vi "Finish.vi"   [LabVIEW 2017]
doc: "This VI is called just before exiting. It is expected to close I/O refnum, save collected data, etc."
uses:
  <vilib>/Rock Robotics/WPI/Utilities/WPI_GetSetVariantRefNum.vi
types:
  T1 = typedef "WPI_MotorControlDeviceRef.ctl" = cluster{"DeviceStatus":errorcluster, "Type":T2, "PWM":cluster{"PWM Channel":T3, "DeadBand":T4}, "CAN":cluster{"Device Number":u8, "SetOutput VI Ref":variant, "GetOutput VI Ref":variant, "Enable VI Ref":variant, "Disable VI Ref":variant, "Data":variant}, "Invert":bool, "DIO PWM":cluster{"PWM \"Enable\" Channel":T3, "DIOChannel":T5, "PWM Rate":dbl}}
  T2 = typedef "WPI_MotorControlType.ctl" = enum16{"PWM", "CAN", "DIO PWM"}
  T3 = typedef "FPGA_DIOPWMChannel.ctl" = enum8{"PWM 0", "PWM 1", "PWM 2", "PWM 3", "PWM 4", "PWM 5", "PWM 6", "PWM 7", "PWM 8", "PWM 9", "PWM MXP 0", "PWM MXP 1", "PWM MXP 2", "PWM MXP 3", "PWM MXP 4", "PWM MXP 5", "PWM MXP 6", "PWM MXP 7", "PWM MXP 8", "PWM MXP 9", "Invalid"}
  T4 = typedef "WPI_PWMDeadband.ctl" = cluster{"Name":string, "maxPositivePwm":i32, "minPositivePwm":i32, "centerPwm":i32, "maxNegativePwm":i32, "minNegativePwm":i32, "angularRange":u16}
  T5 = typedef "FPGA_DIOChannel.ctl" = enum8{"DIO 0", "DIO 1", "DIO 2", "DIO 3", "DIO 4", "DIO 5", "DIO 6", "DIO 7", "DIO 8", "DIO 9", "DIO MXP 0", "DIO MXP 1", "DIO MXP 2", "DIO MXP 3", "DIO MXP 4", "DIO MXP 5", "DIO MXP 6", "DIO MXP 7", "DIO MXP 8", "DIO MXP 9", "DIO MXP 10", "DIO MXP 11", "DIO MXP 12", "DIO MXP 13", "DIO MXP 14", "DIO MXP 15", "SPI Port CS1", "SPI Port CS2", "SPI Port CS3", "SPI Port MISO", "SPI Port MOSI", "Invalid"}
  T6 = typedef "WPI_CompressorDevRef.ctl" = cluster{"DevStatus":errorcluster, "Pneumatics Control Module":u8}
  T7 = typedef "WPI_JoystickDevRef.ctl" = cluster{"Device":T8}
  T8 = typedef "WPI_JoystickDeviceEnum.ctl" = enum16{"USB 0", "USB 1", "USB 2", "USB 3", "USB 4", "USB 5"}
  T9 = typedef "WPI_SolenoidDevRef.ctl" = cluster{"DevStatus":errorcluster, "Pneumatics Control Module":u8, "Forward Solenoid Channel":T10, "Reverse Solenoid Channel":T10}
  T10 = typedef "WPI_SolenoidChannel.ctl" = enum8{"Solenoid 0", "Solenoid 1", "Solenoid 2", "Solenoid 3", "Solenoid 4", "Solenoid 5", "Solenoid 6", "Solenoid 7", "Invalid"}
  T11 = typedef "WPI_EncoderDevRef.ctl" = cluster{"DevStatus":errorcluster, "EncoderIndex":T12, "CounterIndex":T13, "DistancePerCount":dbl, "Decoding Type":T14}
  T12 = typedef "FPGA_EncoderIdx.ctl" = enum8{"Enc 0", "Enc 1", "Enc 2", "Enc 3", "Enc 4", "Enc 5", "Enc 6", "Enc 7", "Invalid"}
  T13 = typedef "FPGA_CounterCtrSystemIndex.ctl" = enum8{"Ctr 0", "Ctr 1", "Ctr 2", "Ctr 3", "Ctr 4", "Ctr 5", "Ctr 6", "Ctr 7", "Invalid"}
  T14 = typedef "WPI_EncoderType.ctl" = enum16{"1x", "2x", "4x"}
  T15 = typedef "WPI_SwitchDevRef.ctl" = cluster{"DevStatus":errorcluster, "DIO Channel":T5, "CntIndex":T13, "Normally Closed":bool}
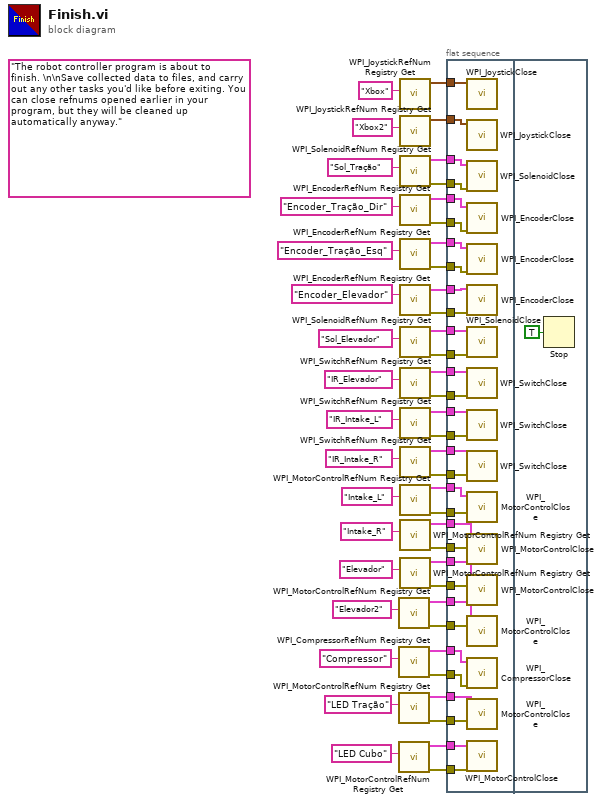
[diagram p0: block diagram]
diagram:
  (unwired) "The robot controller program is about to finish. \n\nSave collected data to files, and carry out any other tasks you'd like before exiting. You can close refnums opened earlier in your program, but they will be cleaned up automatically anyway."
  n1 = call <vilib>:"WPI_MotorControlRefNum Registry Get.vi"("refnum name"="Elevador2") -> ("error out"=w10:errorcluster, "MotorControlDevRef"=w11:T1)  [unwired: 9 in]
  n2 = call <vilib>:"WPI_CompressorRefNum Registry Get.vi"("refnum name"="Compressor") -> ("error out"=w7:errorcluster, "CompressorDevRef"=w8:T6)  [unwired: 9 in]
  n3 = call <vilib>:"WPI_MotorControlRefNum Registry Get.vi"("refnum name"="LED Tração") -> ("error out"=w3:errorcluster, "MotorControlDevRef"=w4:T1)  [unwired: 9 in]
  n4 = call <vilib>:"WPI_MotorControlRefNum Registry Get.vi"("refnum name"="LED Cubo") -> ("error out"=w1:errorcluster, "MotorControlDevRef"=w2:T1)  [unwired: 9 in]
  n5 = call <vilib>:"WPI_JoystickRefNum Registry Get.vi"("refnum name"="Xbox") -> ("JoystickDevRef"=w49:T7)  [unwired: 9 in, 1 out]
  n6 = call <vilib>:"WPI_JoystickRefNum Registry Get.vi"("refnum name"="Xbox2") -> ("JoystickDevRef"=w48:T7)  [unwired: 9 in, 1 out]
  n7 = call <vilib>:"WPI_SolenoidRefNum Registry Get.vi"("refnum name"="Sol_Tração") -> ("error out"=w44:errorcluster, "SolenoidDevRef"=w45:T9)  [unwired: 9 in]
  n8 = call <vilib>:"WPI_EncoderRefNum Registry Get.vi"("refnum name"="Encoder_Tração_Dir") -> ("error out"=w41:errorcluster, "EncoderDevRef"=w42:T11)  [unwired: 9 in]
  n9 = call <vilib>:"WPI_EncoderRefNum Registry Get.vi"("refnum name"="Encoder_Tração_Esq") -> ("error out"=w17:errorcluster, "EncoderDevRef"=w16:T11)  [unwired: 9 in]
  n10 = call <vilib>:"WPI_EncoderRefNum Registry Get.vi"("refnum name"="Encoder_Elevador") -> ("error out"=w14:errorcluster, "EncoderDevRef"=w15:T11)  [unwired: 9 in]
  n11 = call <vilib>:"WPI_SolenoidRefNum Registry Get.vi"("refnum name"="Sol_Elevador") -> ("error out"=w39:errorcluster, "SolenoidDevRef"=w38:T9)  [unwired: 9 in]
  n12 = call <vilib>:"WPI_SwitchRefNum Registry Get.vi"("refnum name"="IR_Elevador") -> ("error out"=w35:errorcluster, "SwitchDevRef"=w36:T15)  [unwired: 9 in]
  n13 = call <vilib>:"WPI_SwitchRefNum Registry Get.vi"("refnum name"="IR_Intake_L") -> ("error out"=w33:errorcluster, "SwitchDevRef"=w32:T15)  [unwired: 9 in]
  n14 = call <vilib>:"WPI_SwitchRefNum Registry Get.vi"("refnum name"="IR_Intake_R") -> ("error out"=w30:errorcluster, "SwitchDevRef"=w31:T15)  [unwired: 9 in]
  n15 = call <vilib>:"WPI_MotorControlRefNum Registry Get.vi"("refnum name"="Intake_L") -> ("error out"=w26:errorcluster, "MotorControlDevRef"=w27:T1)  [unwired: 9 in]
  n16 = call <vilib>:"WPI_MotorControlRefNum Registry Get.vi"("refnum name"="Intake_R") -> ("error out"=w25:errorcluster, "MotorControlDevRef"=w24:T1)  [unwired: 9 in]
  n17 = call <vilib>:"WPI_MotorControlRefNum Registry Get.vi"("refnum name"="Elevador") -> ("error out"=w21:errorcluster, "MotorControlDevRef"=w20:T1)  [unwired: 9 in]
  n18 = flat-sequence {
    tunnel: w49 -> [w81]
    tunnel: w48 -> [w80]
    tunnel: w45 -> [w79]
    tunnel: w44 -> [w78]
    tunnel: w42 -> [w77]
    tunnel: w41 -> [w76]
    tunnel: w38 -> [w74]
    tunnel: w39 -> [w75]
    tunnel: w36 -> [w73]
    tunnel: w35 -> [w72]
    tunnel: w32 -> [w70]
    tunnel: w33 -> [w71]
    tunnel: w31 -> [w69]
    tunnel: w30 -> [w68]
    tunnel: w27 -> [w67]
    tunnel: w26 -> [w66]
    tunnel: w25 -> [w65]
    tunnel: w24 -> [w64]
    tunnel: w21 -> [w63]
    tunnel: w20 -> [w62]
    tunnel: w16 -> [w60]
    tunnel: w17 -> [w61]
    tunnel: w15 -> [w59]
    tunnel: w14 -> [w58]
    tunnel: w10 -> [w56]
    tunnel: w11 -> [w57]
    tunnel: w8 -> [w55]
    tunnel: w7 -> [w54]
    tunnel: w4 -> [w53]
    tunnel: w3 -> [w52]
    tunnel: w2 -> [w51]
    tunnel: w1 -> [w50]
    frame #0 {
      n19 = call <vilib>:"WPI_JoystickClose.vi"("JoystickDevRef"=w81) -> ()  [unwired: 11 in]
      n20 = call <vilib>:"WPI_JoystickClose.vi"("JoystickDevRef"=w80) -> ()  [unwired: 11 in]
      n21 = call <vilib>:"WPI_SolenoidClose.vi"("error in (no error)"=w78, "SolenoidDevRef"=w79) -> ()  [unwired: 9 in, 1 out]
      n22 = call <vilib>:"WPI_EncoderClose.vi"("error in (no error)"=w76, "EncoderDevRef"=w77) -> ()  [unwired: 9 in, 1 out]
      n23 = call <vilib>:"WPI_EncoderClose.vi"("error in (no error)"=w61, "EncoderDevRef"=w60) -> ()  [unwired: 9 in, 1 out]
      n24 = call <vilib>:"WPI_EncoderClose.vi"("error in (no error)"=w58, "EncoderDevRef"=w59) -> ()  [unwired: 9 in, 1 out]
      n25 = call <vilib>:"WPI_SolenoidClose.vi"("error in (no error)"=w75, "SolenoidDevRef"=w74) -> ()  [unwired: 9 in, 1 out]
      n26 = call <vilib>:"WPI_SwitchClose.vi"("error in (no error)"=w72, "SwitchDevRef"=w73) -> ()  [unwired: 9 in, 1 out]
      n27 = call <vilib>:"WPI_SwitchClose.vi"("error in (no error)"=w71, "SwitchDevRef"=w70) -> ()  [unwired: 9 in, 1 out]
      n28 = call <vilib>:"WPI_SwitchClose.vi"("error in (no error)"=w68, "SwitchDevRef"=w69) -> ()  [unwired: 9 in, 1 out]
      n29 = call <vilib>:"WPI_MotorControlClose.vi"("error in"=w66, "MotorControlDevRef"=w67) -> ()  [unwired: 9 in, 1 out]
      n30 = call <vilib>:"WPI_MotorControlClose.vi"("error in"=w65, "MotorControlDevRef"=w64) -> ()  [unwired: 9 in, 1 out]
      n31 = call <vilib>:"WPI_MotorControlClose.vi"("error in"=w63, "MotorControlDevRef"=w62) -> ()  [unwired: 9 in, 1 out]
      n32 = call <vilib>:"WPI_MotorControlClose.vi"("error in"=w56, "MotorControlDevRef"=w57) -> ()  [unwired: 9 in, 1 out]
      n33 = call <vilib>:"WPI_CompressorClose.vi"("error in (no error)"=w54, "CompressorDevRef"=w55) -> ()  [unwired: 9 in, 1 out]
      n34 = call <vilib>:"WPI_MotorControlClose.vi"("error in"=w52, "MotorControlDevRef"=w53) -> ()  [unwired: 9 in, 1 out]
      n35 = call <vilib>:"WPI_MotorControlClose.vi"("error in"=w50, "MotorControlDevRef"=w51) -> ()  [unwired: 9 in, 1 out]
    }
    frame #1 {
      n36 = Stop(stop? (T)=TRUE ("Quit")) -> ()
    }
  }
